vi "1 Sync - Software Trigger.vi"() -> ()   [LabVIEW 2023]
doc: "This example demonstrates how to acquire a single buffer of voltage measurements using a DAQmx device.\n\nFor instructions on how to connect your signals to the DAQ device, refer to your device documentation."
uses:
  <vilib>/DAQmx/create/channels.llb/DAQmx Create Channel (AI-Voltage-Basic).vi
  <vilib>/DAQmx/configure/timing.llb/DAQmx Timing (Sample Clock).vi
  <vilib>/DAQmx/read.llb/DAQmx Read (Analog Wfm 1Chan NSamp).vi
  <vilib>/Analysis/NI_AALBase.lvlib
  <resource>/objmgr/daqmx.rc
  <vilib>/DAQmx/configure/timing.llb/DAQmx Timing (Implicit).vi
  <vilib>/DAQmx/create/channels.llb/DAQmx Create Channel (CO-Pulse Generation-Frequency).vi
panel:
  in  "Square Wave Output: Terminal":tag="/MIODAQ/PFI0"
  in  "Square Wave Output: Source":tag="MIODAQ/ctr0"
  out "Progress":i32(slide) scale=0.0..9.0
  out "Standard Deviation":dbl format="%0.2f"
  out "Range":dbl
  out "Mean":dbl format="%0.2f"
  out "Skew":dbl
  in  "Device 2: Analog Input Channel":tag="cDAQ9189-2628AACMod1/ai0"
  out "Waveform Graph":waveform(dbl)[](graph)
  in  "Device 1: Analog Input Channel":tag="MIODAQ/ai0"
  # "Channel Settings"
  # "Acquired Data"
  # "Output Signal Settings"
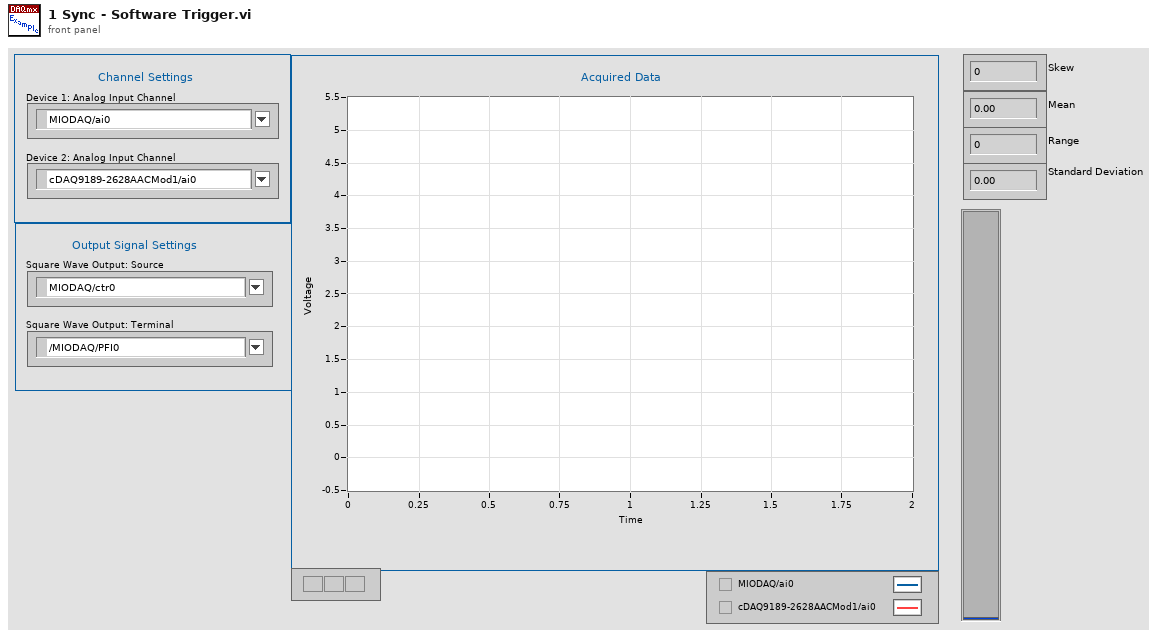
[diagram p1: front panel]
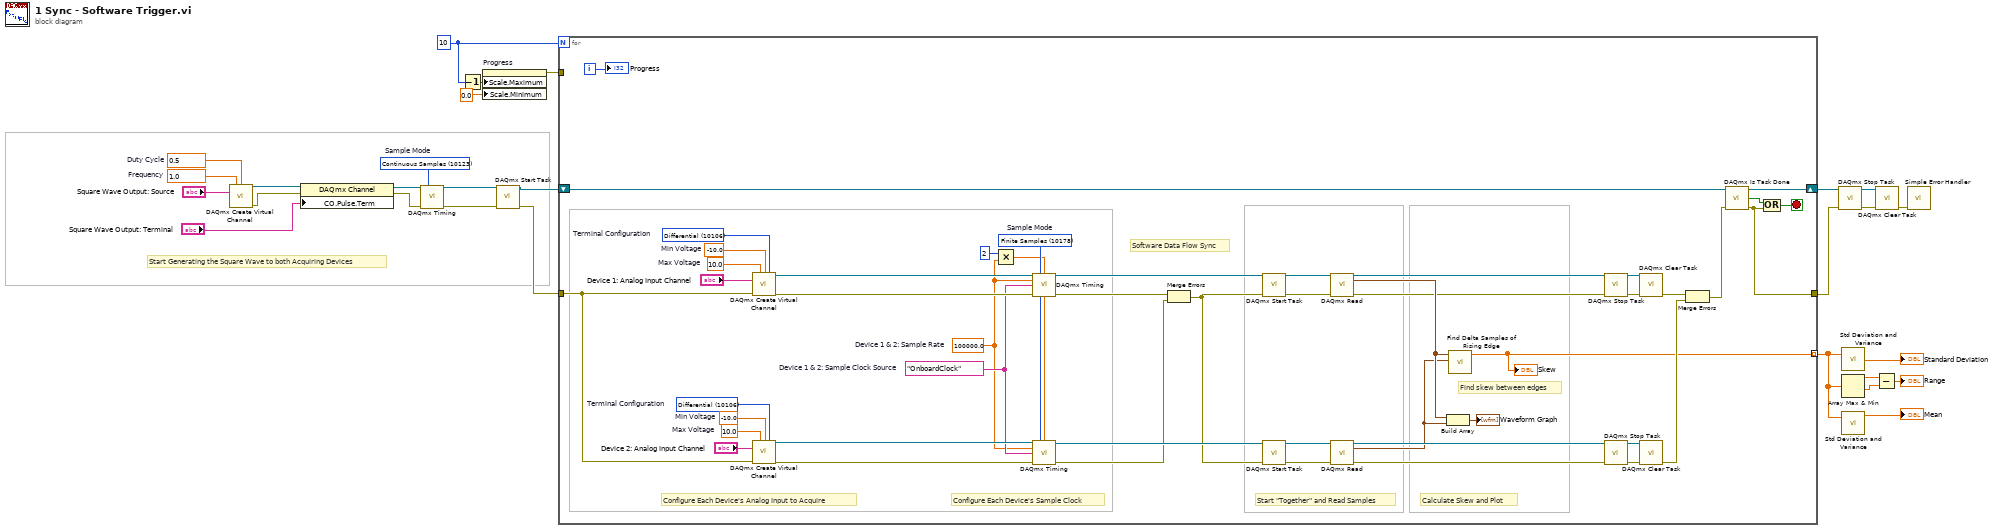
[diagram p0: block diagram]
diagram:
  w16 = 1.0  # Frequency
  w17 = 0.5  # Duty Cycle
  w9 = 10123 items=["Finite Samples"=10178, "Continuous Samples"=10123, "Hardware Timed Single Point"=12522]  # Sample Mode
  w22 = 10
  # "Start Generating the Square Wave to both Acquiring Devices"
  n1 = call-poly <vilib>:"DAQmx Create Virtual Channel.vi"("frequency"=w16, "duty cycle"=w17, "counter"="Square Wave Output: Source") -> ("task out"=w11:refnum<k21>, "error out"=w12:errorcluster)  [unwired: 11 in]
  n2 = property class="DAQmx Channel"(reference=w11, error in=w12, "CO.Pulse.Term"="Square Wave Output: Terminal") -> (reference out=w15:refnum<k21>, error out=w14:errorcluster)
  n3 = call-poly <vilib>:"DAQmx Timing.vi"("task/channels in"=w15, "sample mode"=w9, "error in"=w14) -> ("task out"=w19:refnum<k21>, "error out"=w18:errorcluster)  [unwired: 11 in]
  n4 = Decrement(x=w22) -> (x-1=w1:i32)
  n5 = property on="Progress" class="Slide (strict)"("Scale.Maximum"=w1, "Scale.Minimum"=0.0 ("Scale.Range:Minimum")) -> (error out=w20:errorcluster)  [unwired: 2 in, 1 out]
  n6 = call <vilib>:"DAQmx Start Task.vi"("task/channels in"=w19, "error in"=w18) -> ("task out"=w5:refnum<k21>, "error out"=w6:errorcluster)  [unwired: 12 in]
  n7 = for {
    N: w22 -> [_]
    tunnel: [w30] -> w24 mode=indexing
    tunnel: w20 -> [_]
    tunnel: [w38] -> w3
    tunnel: w6 -> [w29]
    shift-right: [w35] -> w4
    shift-left: w5 -> [w34]
    i -> [w47]
    stop <- w36 stop-if-true
    w33 = 100000.0  # Device 1 & 2: Sample Rate
    w58 = tag "OnboardClock"  # Device 1 & 2: Sample Clock Source
    w64 = 10.0  # Max Voltage
    w63 = -10.0  # Min Voltage
    w62 = 10106 items=["default"=-1, "RSE"=10083, "NRSE"=10078, "Differential"=10106, "Pseudodifferential"=12529]  # Terminal Configuration
    w68 = 10.0  # Max Voltage
    w69 = -10.0  # Min Voltage
    w70 = 10106 items=["default"=-1, "RSE"=10083, "NRSE"=10078, "Differential"=10106, "Pseudodifferential"=12529]  # Terminal Configuration
    w46 = 10178 items=["Finite Samples"=10178, "Continuous Samples"=10123, "Hardware Timed Single Point"=12522]  # Sample Mode
    # "Calculate Skew and Plot"
    # "Start \"Together\" and Read Samples"
    # "Software Data Flow Sync"
    # "Configure Each Device's Sample Clock"
    # "Configure Each Device's Analog Input to Acquire"
    # "Find skew between edges"
    n8 = call-poly <vilib>:"DAQmx Create Virtual Channel.vi"("maximum value"=w68, "minimum value"=w69, "input terminal configuration"=w70, "physical channels"="Device 1: Analog Input Channel", "error in"=w29) -> ("task out"=w74:refnum<k21>, "error out"=w75:errorcluster)  [unwired: 9 in]
    n9 = call-poly <vilib>:"DAQmx Create Virtual Channel.vi"("maximum value"=w64, "minimum value"=w63, "input terminal configuration"=w62, "physical channels"="Device 2: Analog Input Channel", "error in"=w29) -> ("task out"=w61:refnum<k21>, "error out"=w60:errorcluster)  [unwired: 9 in]
    n10 = Multiply(x=2, y=w33) -> (x*y=w31:dbl)
    n11 = call-poly <vilib>:"DAQmx Timing.vi"("task/channels in"=w74, "sample mode"=w46, "samples per channel"=w31, "rate"=w33, "source"=w58, "error in"=w75) -> ("task out"=w76:refnum<k21>, "error out"=w45:errorcluster)  [unwired: 8 in]
    n12 = call-poly <vilib>:"DAQmx Timing.vi"("task/channels in"=w61, "sample mode"=w46, "samples per channel"=w31, "rate"=w33, "source"=w58, "error in"=w60) -> ("task out"=w51:refnum<k21>, "error out"=w44:errorcluster)  [unwired: 8 in]
    n13 = Merge Errors(w45, w44) -> (w43:errorcluster)
    n14 = call <vilib>:"DAQmx Start Task.vi"("task/channels in"=w76, "error in"=w43) -> ("task out"=w73:refnum<k21>, "error out"=w72:errorcluster)  [unwired: 12 in]
    n15 = call <vilib>:"DAQmx Start Task.vi"("task/channels in"=w51, "error in"=w43) -> ("task out"=w52:refnum<k21>, "error out"=w53:errorcluster)  [unwired: 12 in]
    n16 = call-poly <vilib>:"DAQmx Read.vi"("task/channels in"=w73, "error in"=w72) -> ("task out"=w65:refnum<k21>, "data"=w49:waveform(dbl), "error out"=w40:errorcluster)  [unwired: 11 in]
    n17 = call-poly <vilib>:"DAQmx Read.vi"("task/channels in"=w52, "error in"=w53) -> ("task out"=w56:refnum<k21>, "data"=w48:waveform(dbl), "error out"=w57:errorcluster)  [unwired: 11 in]
    n18 = Build Array(w49, w48) -> (→"Waveform Graph":waveform(dbl)[])
    n19 = call "Find Delta Samples of Rising Edge.vi"("Channel 2"=w48, "Channel 1"=w49) -> ("Sample Offset"=w30:dbl)  [unwired: 9 in]
    "Skew" <- w30
    n20 = call <vilib>:"DAQmx Stop Task.vi"("task/channels in"=w65, "error in"=w40) -> ("task out"=w67:refnum<k21>, "error out"=w66:errorcluster)  [unwired: 12 in]
    n21 = call <vilib>:"DAQmx Stop Task.vi"("task/channels in"=w56, "error in"=w57) -> ("task out"=w54:refnum<k21>, "error out"=w55:errorcluster)  [unwired: 12 in]
    n22 = call <vilib>:"DAQmx Clear Task.vi"("task in"=w67, "error in"=w66) -> ("error out"=w41:errorcluster)  [unwired: 13 in]
    n23 = call <vilib>:"DAQmx Clear Task.vi"("task in"=w54, "error in"=w55) -> ("error out"=w42:errorcluster)  [unwired: 13 in]
    n24 = Merge Errors(w41, w42) -> (w39:errorcluster)
    n25 = call <vilib>:"DAQmx Is Task Done.vi"("task/channels in"=w34, "error in"=w39) -> ("task out"=w35:refnum<k21>, "task done?"=w37:bool, "error out"=w38:errorcluster)  [unwired: 11 in]
    n26 = Compound Arithmetic op=OR(w37, w38) -> (w36:bool)
    "Progress" <- w47
  }
  n27 = call <vilib>:"DAQmx Stop Task.vi"("task/channels in"=w4, "error in"=w3) -> ("task out"=w7:refnum<k21>, "error out"=w8:errorcluster)  [unwired: 12 in]
  n28 = call <vilib>:"Std Deviation and Variance.vi"("X"=w24) -> ("standard deviation"=→"Standard Deviation":dbl)  [unwired: 1 in, 2 out]
  n29 = Array Max & Min(array=w24) -> (max value=w28:dbl, min value=w27:dbl)  [unwired: 2 out]
  n30 = call <vilib>:"Std Deviation and Variance.vi"("X"=w24) -> ("mean"=→"Mean":dbl)  [unwired: 1 in, 2 out]
  n31 = Subtract(x=w28, y=w27) -> (x-y=→"Range":dbl)
  n32 = call <vilib>:"DAQmx Clear Task.vi"("task in"=w7, "error in"=w8) -> ("error out"=w2:errorcluster)  [unwired: 13 in]
  n33 = call <vilib>:"Simple Error Handler.vi"("error in (no error)"=w2) -> ()  [unwired: 4 in, 5 out]
